vi "Main.vi"(8 "Error In":errorcluster) -> (0 "Error Out":errorcluster)   [LabVIEW 2017, in "Processing.lvlib"]
uses:
  Processing.lvlib
  Controls/Commands [enum].ctl
  File IO/Controls/Params.ctl
  System Control/CTLs/Test params.ctl
  System Control/CTLs/Test Controls.ctl
  System Control/CTLs/Test indicators.ctl
  System Control/CTLs/Test Type.ctl
  Events/Controls/Action Refs [enum].ctl
  System Control/Main controller.lvlib
  Events/Events.lvlib
  File IO/File IO.lvlib
  UI/UI.lvlib
panel:
  in  "Test":T1={"Config"={"Amplification Factor"=2.0, "100% Reflectance Standard"=2.0, "Calculation Method"=enum."Reflectance", "Option to discard new data?"=FALSE, "Mode"=enum."Spectrum", "Number of Averages"=0, "B Test?"=FALSE}, "Indicators"={"DAQ Background Level (V)"=2.0, "A-Test Counter"=2, "B-Test Counter"=2, "Type"=enum."A-Test", "Scope Background Level (Amps)"=2.0, "TAS only?"=FALSE}} {"Config"."Number of Averages" min=0}
  in  "File IO parameters":T5={"Output Folder"=path "C:/Users/Abigail/Documents/Imperial Optical software/Optical Software Code Simplified/Output", "Error file"=path "Error Log.txt", "Config file"=path "Config.ini", "File prefix"="", "Waveform read"={"t0"=timestamp(0 s since 1904-01-01), "dt"=1.0, "Y"=[]}}
  in  "Change state":T6
  out "Standalone":bool=TRUE
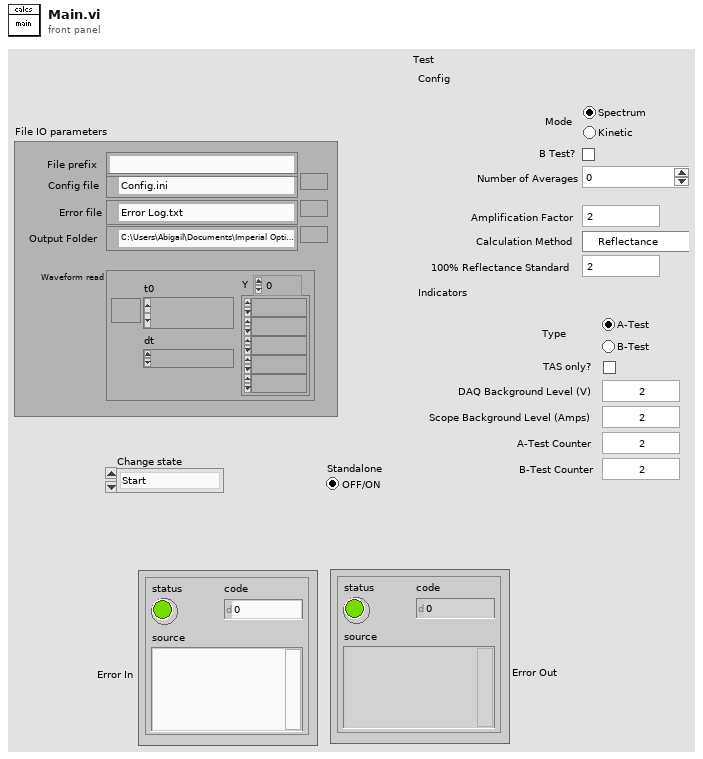
[diagram p1: front panel]
types:
  T1 = typedef "Main controller.lvlib/Test params.ctl" = cluster{"Config":T2, "Indicators":T3}
  T2 = typedef "Main controller.lvlib/Test Controls.ctl" = cluster{"Amplification Factor":dbl, "100% Reflectance Standard":dbl, "Calculation Method":enum16{"Reflectance", "Transmission", "Kubelka-Munk"}, "Option to discard new data?":bool, "Mode":enum32{"Spectrum", "Kinetic"}, "Number of Averages":i32, "B Test?":bool}
  T3 = typedef "Main controller.lvlib/Test indicators.ctl" = cluster{"DAQ Background Level (V)":dbl, "A-Test Counter":i32, "B-Test Counter":i32, "Type":T4, "Scope Background Level (Amps)":dbl, "TAS only?":bool}
  T4 = typedef "Main controller.lvlib/Test Type.ctl" = enum32{"A-Test", "B-Test"}
  T5 = typedef "File IO.lvlib/Params.ctl" = cluster{"Output Folder":path, "Error file":path, "Config file":path, "File prefix":string, "Waveform read":waveform(dbl)}
  T6 = typedef "Processing.lvlib/Commands [enum].ctl" = enum16{"Start", "Stop", "Process waveform", "Scope A-B processing", "DAQ A-B processing", "DAQ-Scope Stitching", "Update Test Info"}
  T7 = enum32{"Bad", "Idle", "Run top level", "Running"}
  T8 = typedef "Events.lvlib/Action Refs [enum].ctl" = enum16{"Init", "Ref", "Kill"}
  T9 = typedef "Events.lvlib/Refs [cluster].ctl" = cluster{"Exit":refnum<user-event>, "Controller":refnum<user-event>, "System Error":refnum<user-event>, "UI":refnum<user-event>, "Example Module":refnum<user-event>, "Shutter":refnum<user-event>, "Monochromator":refnum<user-event>, "DAQ":refnum<user-event>, "Scope":refnum<user-event>, "Processing":refnum<user-event>, "File IO":refnum<user-event>, "Colour wheel":refnum<user-event>}
  T10 = cluster{"Debug Waveform Read":dbl[][], "Waveform name":string}
  T11 = cluster{"File IO":T5, "Filename (A)":string, "Filename (B)":string}
  T12 = cluster{"File IO":T5, "DAQ Filename":string, "Scope Filename":string}
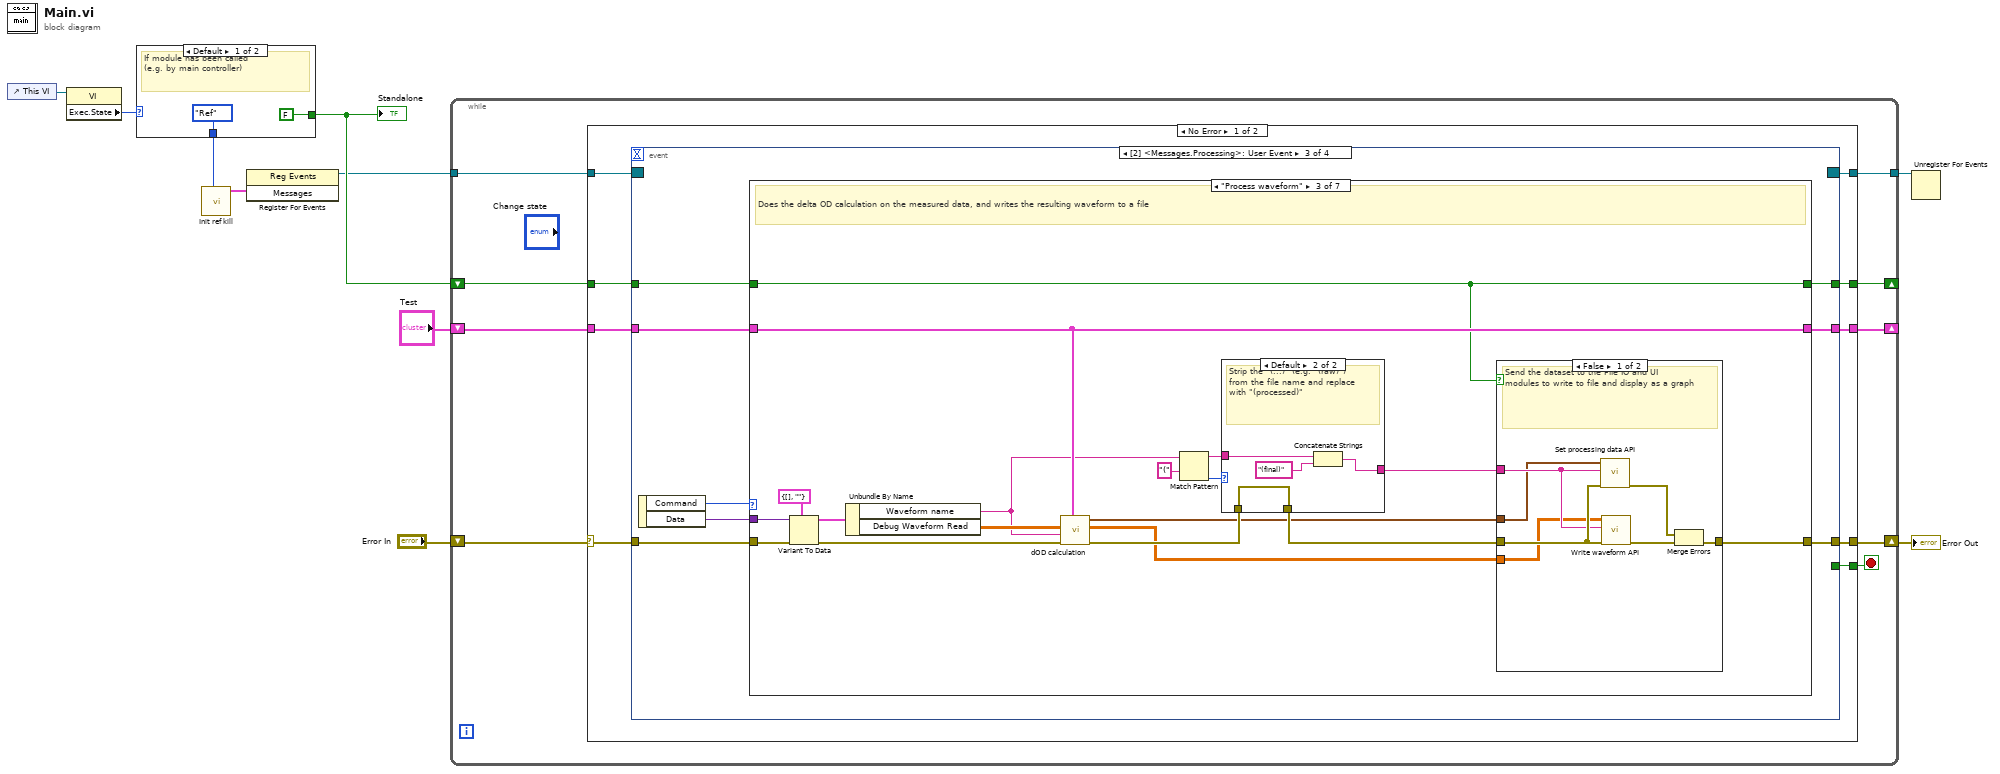
[diagram p0: block diagram]
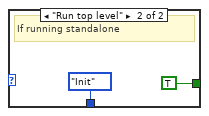
[diagram p2: hidden frame]
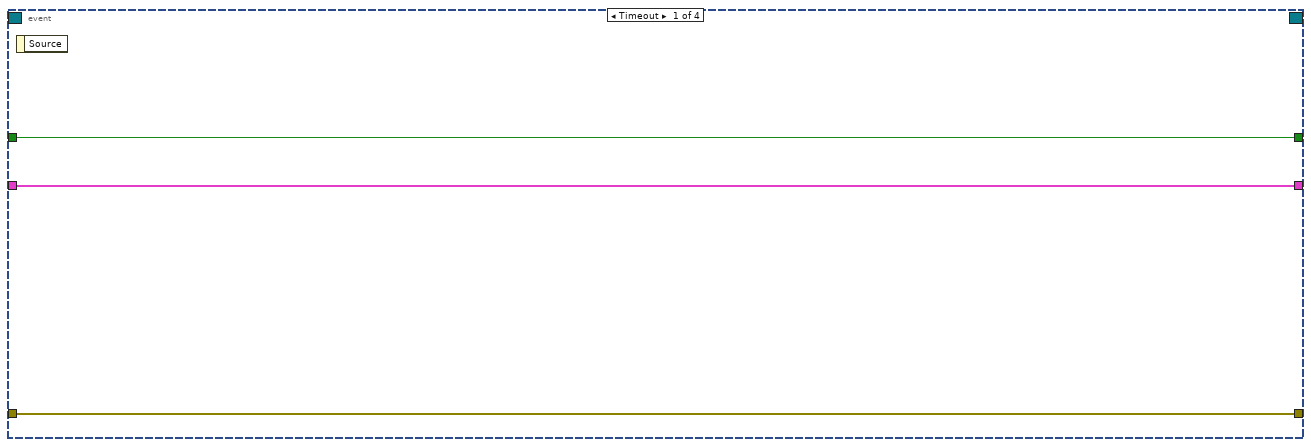
[diagram p3: hidden frame]
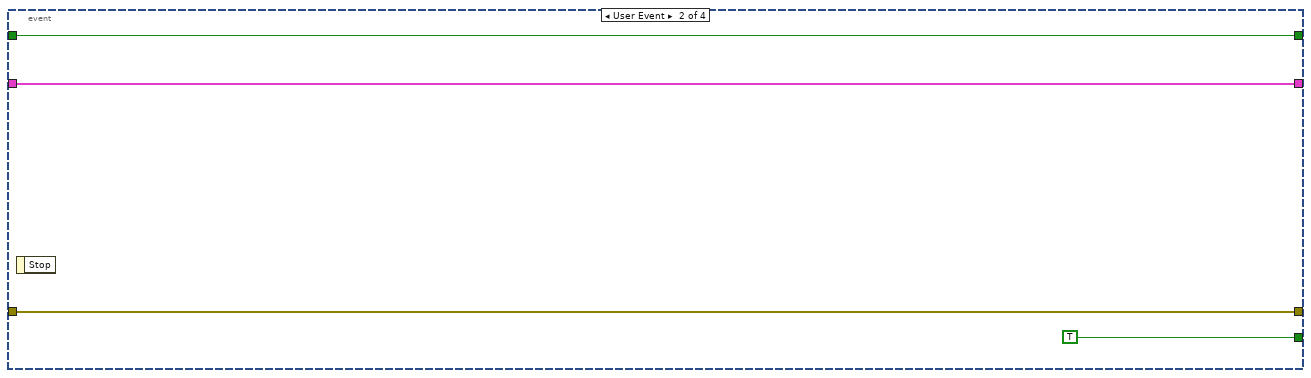
[diagram p4: hidden frame]
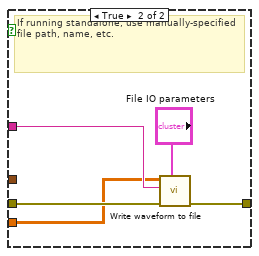
[diagram p7: hidden frame]
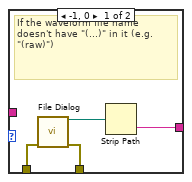
[diagram p8: hidden frame]
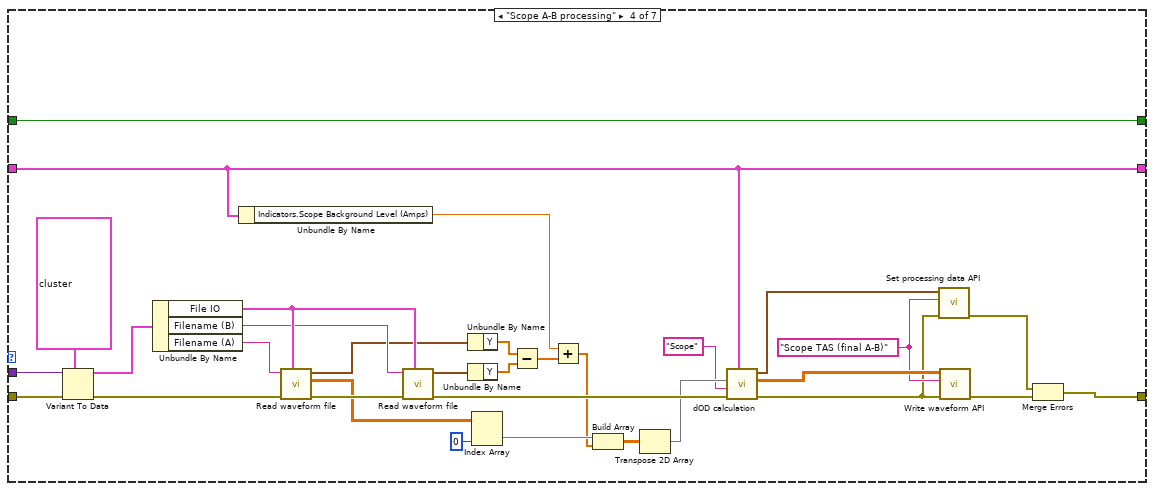
[diagram p9: hidden frame]
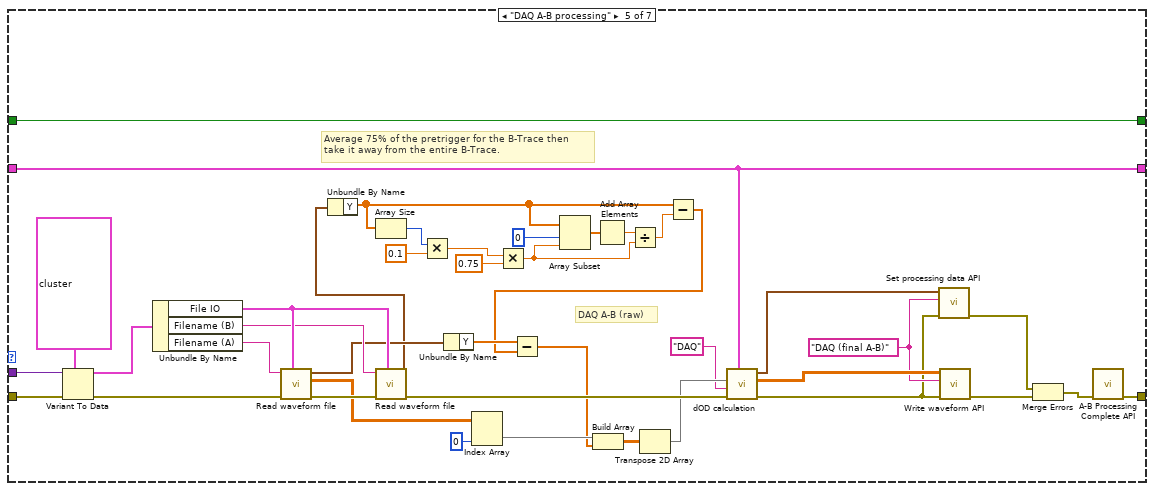
[diagram p10: hidden frame]
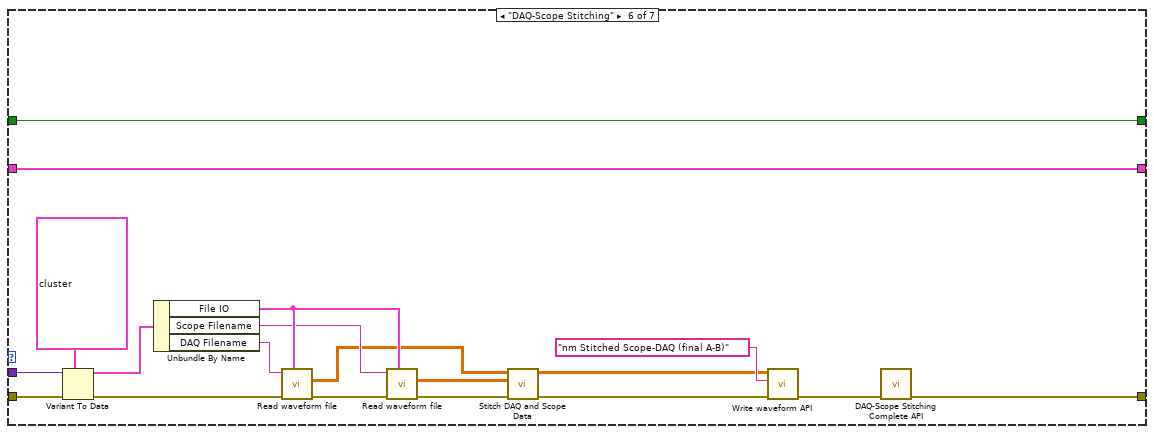
[diagram p11: hidden frame]
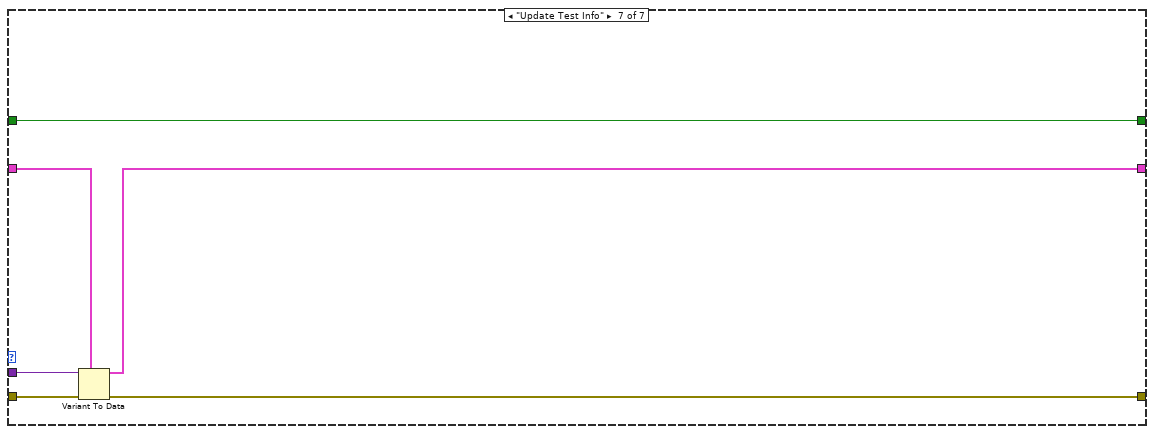
[diagram p12: hidden frame]
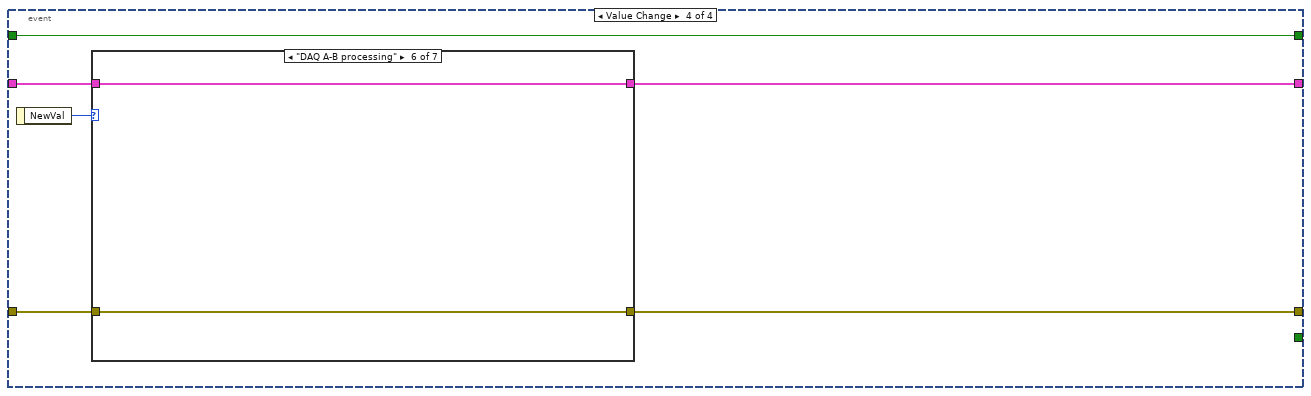
[diagram p13: hidden frame]
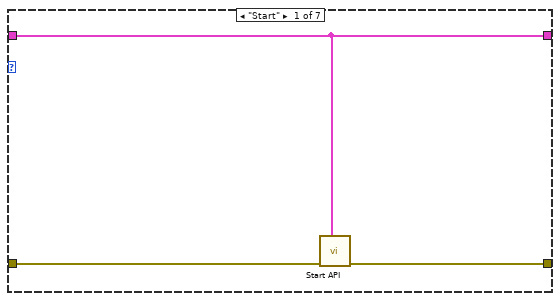
[diagram p14: hidden frame]
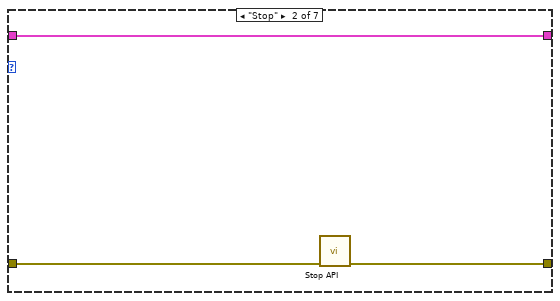
[diagram p15: hidden frame]
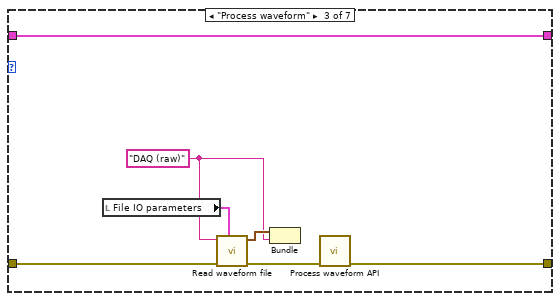
[diagram p16: hidden frame]
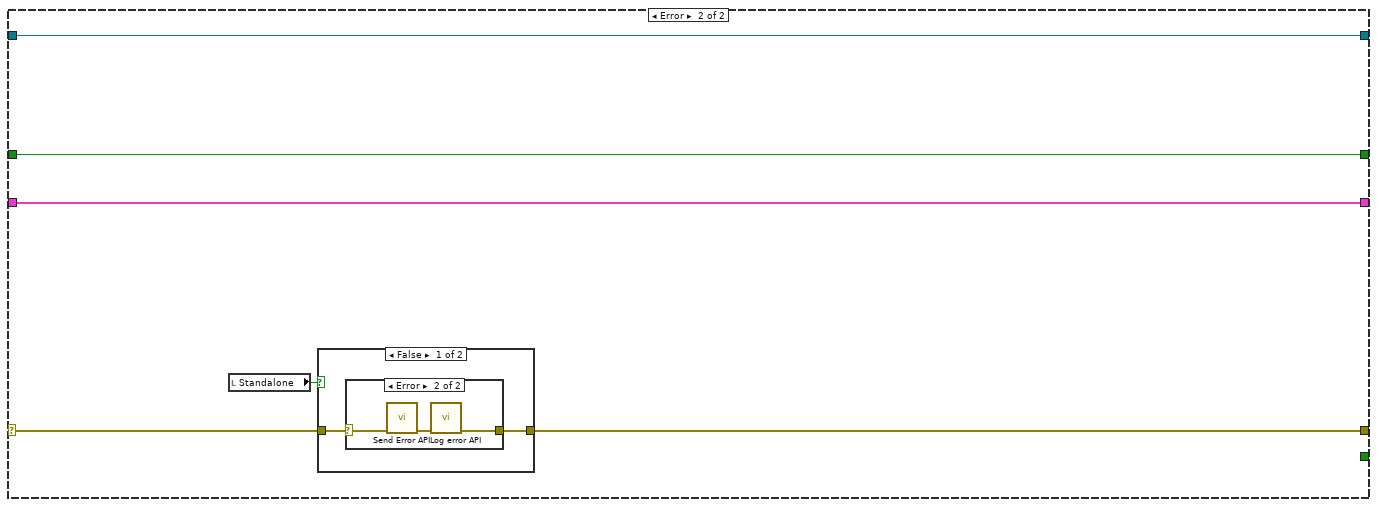
[diagram p20: hidden frame]
diagram:
  n1 = control-ref of="This VI"() -> (w5:refnum<vi>)
  n2 = property class="VI"(reference=w5) -> ("Exec.State"=w4:T7)  [unwired: 1 in, 2 out]
  n3 = case shown="Default" w4 {
    tunnel: [Action_Refs_[enum]."Ref" ("Action") Action_Refs_[enum]."Init" ("Action")] -> w3
    tunnel: [FALSE TRUE] -> w2
    frame Default {
      # "If module has been called\n(e.g. by main controller)"
    }
    frame "Run top level" {
      # "If running standalone"
    }
  }
  "Standalone" <- w2
  n4 = call "Init ref kill.vi"("Action"=w3) -> ("Messages"=w6:T9)  [unwired: 9 in, 1 out]
  n5 = register-events(w6) -> (reference out=w1:refnum<event-registration>)  [unwired: 2 in, 1 out]
  n6 = while {
    tunnel: w1 -> [w23]
    shift-right: [w20] -> _
    shift-left: w2 -> [w19]
    tunnel: [w21] -> w10
    shift-right: [w16] -> w8
    shift-left: "Error In" -> [w15]
    shift-right: [w17] -> _
    shift-left: "Test" -> [w18]
    stop <- w22 stop-if-true
    n7 = case shown="No Error" w15 {
      selector: w15 -> [w24 w222]
      tunnel: w23 -> [w32 w217]
      tunnel: [w31 _] -> w22
      tunnel: [w30 w217] -> w21
      tunnel: [w29 w218] -> w20
      tunnel: w19 -> [w28 w218]
      tunnel: w18 -> [w27 w219]
      tunnel: [w26 w219] -> w17
      tunnel: [w25 w221] -> w16
      frame No Error {
        n8 = event shown="[2] <Messages.Processing>: User Event" {
          selector: w32 -> [_ _ _ _]
          dyn-events: [_ _ _ _] -> w30
          timeout: _ -> [_ _ _ _]
          tunnel: [_ TRUE _ _] -> w31
          tunnel: [w33 w36 w46 w195] -> w29
          tunnel: w28 -> [w33 w36 w45 w195]
          tunnel: w24 -> [w34 w37 w43 w192]
          tunnel: [w34 w37 w42 w191] -> w25
          tunnel: w27 -> [w35 w38 w41 w194]
          tunnel: [w35 w38 w40 w193] -> w26
          event Timeout {
            n9 = event-data() -> ()  [unwired: 1 in, 1 out]
          }
          event User Event {
            n10 = event-data() -> ()  [unwired: 1 in, 1 out]
          }
          event User Event {
            n11 = event-data() -> ("Command"=w47:T6, "Data"=w44:variant)  [unwired: 1 in]
            n12 = case shown="\"Process waveform\"" w47 {
              tunnel: [w49 w52 w59 w123 w164 w183 w189] -> w46
              tunnel: w45 -> [w49 w52 w59 w123 w164 w183 w189]
              tunnel: w44 -> [_ _ w70 w122 w163 w182 w186]
              tunnel: w43 -> [w48 w51 w71 w121 w162 w181 w188]
              tunnel: [w48 w51 w62 w92 w149 w175 w187] -> w42
              tunnel: w41 -> [w50 w53 w63 w94 w137 w178 w185]
              tunnel: [w50 w53 w63 w94 w137 w178 w184] -> w40
              frame "Start" {
                # "Initialise stuff"
              }
              frame "Stop" {
                # "Close stuff"
              }
              frame "Process waveform" {
                # "Does the delta OD calculation on the measured data, and writes the resulting waveform to a file"
                n13 = Variant To Data(error in=w71, type=T10 {"Debug Waveform Read"=[], "Waveform name"=""} ("Waveform + name 2"), Variant=w70) -> (data=w68:T10, error out=w69:errorcluster)
                n14 = Unbundle By Name(w68) -> ("Waveform name"=w54:string, "Debug Waveform Read"=w56:dbl[][])
                n15 = call "dOD calculation.vi"("Test"=w63, "error in"=w69, "Waveform Name"=w54, "Debug Waveform Read In"=w56) -> ("error out"=w64:errorcluster, "Debug Waveform Read Out"=w55:dbl[][], "dOD waveform"=w58:waveform(dbl))  [unwired: 5 in]
                n16 = Match Pattern(string=w54, regular expression="(") -> (before substring=w66:string, offset past match=w65:i32)  [unwired: 1 in, 2 out]
                n17 = case shown="Default" w65 {
                  tunnel: w66 -> [_ w91]
                  tunnel: [w87 w89] -> w60
                  tunnel: w64 -> [w85 w88]
                  tunnel: [w84 w88] -> w61
                  frame -1, 0 {
                    # "If the waveform file name doesn't have \"(...)\" in it (e.g. \"(raw)\")"
                    n18 = call "File Dialog"("error in"=w85) -> ("selected path"=w86:path, "error out"=w84:errorcluster)  [unwired: 11 in, 2 out]
                    n19 = Strip Path(path=w86) -> (name=w87:string)  [unwired: 1 out]
                  }
                  frame Default {
                    # "Strip the \"(...)\" (e.g. \"(raw)\") from the file name and replace with \"(processed)\""
                    n20 = Concatenate Strings(w91, "(final)" ("string")) -> (w89:string)
                  }
                }
                n21 = case shown="False" w59 {
                  tunnel: [w78 w83] -> w62
                  tunnel: w58 -> [w73 _]
                  tunnel: w61 -> [w76 w82]
                  tunnel: w60 -> [w74 w81]
                  tunnel: w55 -> [w72 w79]
                  frame False {
                    # "Send the dataset to the File IO and UI modules to write to file and display as a graph"
                    n22 = call "Set processing data API.vi"("Error In"=w76, "Waveform name"=w74, "Waveform"=w73) -> ("Error Out"=w75:errorcluster)  [unwired: 8 in]
                    n23 = call "Write waveform API.vi"("Error In"=w76, "Waveform name"=w74, "Waveform Data"=w72) -> ("Error Out"=w77:errorcluster)  [unwired: 8 in]
                    n24 = Merge Errors(w75, w77) -> (w78:errorcluster)
                  }
                  frame True {
                    # "If running standalone, use manually-specified file path, name, etc."
                    n25 = call "Write waveform to file.vi"("File IO parameters"="File IO parameters", "error in"=w82, "Dataset name"=w81, "Data"=w79) -> ("error out"=w83:errorcluster)  [unwired: 7 in]
                  }
                }
              }
              frame "Scope A-B processing" {
                w98 = "Scope TAS (final A-B)" ("Waveform name")
                n26 = Variant To Data(error in=w121, type=T11 {"File IO"={"Output Folder"=path "", "Error file"=path "", "Config file"=path "", "File prefix"="", "Waveform read"={"t0"=timestamp(0 s since 1904-01-01), "dt"=1.0, "Y"=[]}}, "Filename (A)"="", "Filename (B)"=""}, Variant=w122) -> (data=w118:T11, error out=w120:errorcluster)
                n27 = Unbundle By Name(w118) -> ("File IO"=w116:T5, "Filename (B)"=w115:string, "Filename (A)"=w114:string)
                n28 = Unbundle By Name(w94) -> ("Indicators.Scope Background Level (Amps)"=w93:dbl)
                n29 = call "Read waveform file.vi"("File IO parameters"=w116, "error in"=w120, "Dataset name"=w114) -> ("error out"=w117:errorcluster, "all rows"=w107:dbl[][], "Waveform"=w113:waveform(dbl))  [unwired: 6 in]
                n30 = call "Read waveform file.vi"("File IO parameters"=w116, "error in"=w117, "Dataset name"=w115) -> ("error out"=w108:errorcluster, "Waveform"=w112:waveform(dbl))  [unwired: 6 in, 1 out]
                n31 = Unbundle By Name(w113) -> ("Y"=w110:dbl[])
                n32 = Unbundle By Name(w112) -> ("Y"=w111:dbl[])
                n33 = Index Array(array=w107, index (col)=0 ("disabled index (col)")) -> (element=w105:dbl[])  [unwired: 1 in]
                n34 = Subtract(x=w110, y=w111) -> (x-y=w109:dbl[])
                n35 = Add(x=w93, y=w109) -> (x+y=w104:dbl[])
                n36 = Build Array(w105, w104) -> (w103:dbl[][])
                n37 = Transpose 2D Array(2D array=w103) -> (transposed array=w102:dbl[][])
                n38 = call "dOD calculation.vi"("Test"=w94, "error in"=w108, "Waveform Name"="Scope", "Debug Waveform Read In"=w102) -> ("error out"=w97:errorcluster, "Debug Waveform Read Out"=w99:dbl[][], "dOD waveform"=w100:waveform(dbl))  [unwired: 5 in]
                n39 = call "Set processing data API.vi"("Error In"=w97, "Waveform name"=w98, "Waveform"=w100) -> ("Error Out"=w96:errorcluster)  [unwired: 8 in]
                n40 = call "Write waveform API.vi"("Error In"=w97, "Waveform name"=w98, "Waveform Data"=w99) -> ("Error Out"=w95:errorcluster)  [unwired: 8 in]
                n41 = Merge Errors(w96, w95) -> (w92:errorcluster)
              }
              frame "DAQ A-B processing" {
                w142 = "DAQ (final A-B)" ("Waveform name")
                # "Average 75% of the pretrigger for the B-Trace then \ntake it away from the entire B-Trace."
                # "DAQ A-B (raw)"
                n42 = Variant To Data(error in=w162, type=T11 {"File IO"={"Output Folder"=path "", "Error file"=path "", "Config file"=path "", "File prefix"="", "Waveform read"={"t0"=timestamp(0 s since 1904-01-01), "dt"=1.0, "Y"=[]}}, "Filename (A)"="", "Filename (B)"=""}, Variant=w163) -> (data=w159:T11, error out=w161:errorcluster)
                n43 = Unbundle By Name(w159) -> ("File IO"=w157:T5, "Filename (B)"=w156:string, "Filename (A)"=w155:string)
                n44 = call "Read waveform file.vi"("File IO parameters"=w157, "error in"=w161, "Dataset name"=w155) -> ("error out"=w158:errorcluster, "all rows"=w151:dbl[][], "Waveform"=w154:waveform(dbl))  [unwired: 6 in]
                n45 = call "Read waveform file.vi"("File IO parameters"=w157, "error in"=w158, "Dataset name"=w156) -> ("error out"=w152:errorcluster, "Waveform"=w125:waveform(dbl))  [unwired: 6 in, 1 out]
                n46 = Unbundle By Name(w125) -> ("Y"=w135:dbl[])
                n47 = Array Size(array=w135) -> (size(s)=w134:i32)
                n48 = Multiply(x=w134, y=0.1) -> (x*y=w133:dbl)
                n49 = Unbundle By Name(w154) -> ("Y"=w153:dbl[])
                n50 = Index Array(array=w151, index (col)=0 ("disabled index (col)")) -> (element=w148:dbl[])  [unwired: 1 in]
                n51 = Multiply(x=w133, y=0.75) -> (x*y=w132:dbl)
                n52 = Array Subset(array=w135, index=0, length=w132) -> (w131:dbl[])
                n53 = Add Array Elements(numeric array=w131) -> (sum=w130:dbl)
                n54 = Divide(x=w130, y=w132) -> (x/y=w129:dbl)
                n55 = Subtract(x=w135, y=w129) -> (x-y=w124:dbl[])
                n56 = Subtract(x=w153, y=w124) -> (x-y=w136:dbl[])
                n57 = Build Array(w148, w136) -> (w147:dbl[][])
                n58 = Transpose 2D Array(2D array=w147) -> (transposed array=w146:dbl[][])
                n59 = call "dOD calculation.vi"("Test"=w137, "error in"=w152, "Waveform Name"="DAQ", "Debug Waveform Read In"=w146) -> ("error out"=w141:errorcluster, "Debug Waveform Read Out"=w143:dbl[][], "dOD waveform"=w144:waveform(dbl))  [unwired: 5 in]
                n60 = call "Set processing data API.vi"("Error In"=w141, "Waveform name"=w142, "Waveform"=w144) -> ("Error Out"=w140:errorcluster)  [unwired: 8 in]
                n61 = call "Write waveform API.vi"("Error In"=w141, "Waveform name"=w142, "Waveform Data"=w143) -> ("Error Out"=w139:errorcluster)  [unwired: 8 in]
                n62 = Merge Errors(w140, w139) -> (w138:errorcluster)
                n63 = call "A-B Processing Complete API.vi"("Error In"=w138) -> ("Error Out"=w149:errorcluster)  [unwired: 10 in]
              }
              frame "DAQ-Scope Stitching" {
                n64 = Variant To Data(error in=w181, type=T12 {"File IO"={"Output Folder"=path "", "Error file"=path "", "Config file"=path "", "File prefix"="", "Waveform read"={"t0"=timestamp(0 s since 1904-01-01), "dt"=1.0, "Y"=[]}}, "DAQ Filename"="", "Scope Filename"=""}, Variant=w182) -> (data=w179:T12, error out=w174:errorcluster)
                n65 = Unbundle By Name(w179) -> ("File IO"=w172:T5, "Scope Filename"=w170:string, "DAQ Filename"=w171:string)
                n66 = call "Read waveform file.vi"("File IO parameters"=w172, "error in"=w174, "Dataset name"=w171) -> ("error out"=w173:errorcluster, "all rows"=w167:dbl[][])  [unwired: 6 in, 1 out]
                n67 = call "Read waveform file.vi"("File IO parameters"=w172, "error in"=w173, "Dataset name"=w170) -> ("error out"=w169:errorcluster, "all rows"=w166:dbl[][])  [unwired: 6 in, 1 out]
                n68 = call "Stitch DAQ and Scope Data.vi"("error in (no error)"=w169, "Scope Ch1 (final A-B)"=w166, "DAQ DOD (final)"=w167) -> ("error out"=w168:errorcluster, "data & time array"=w165:dbl[][])  [unwired: 7 in]
                n69 = call "Write waveform API.vi"("Error In"=w168, "Waveform name"="nm Stitched Scope-DAQ (final A-B)", "Waveform Data"=w165) -> ("Error Out"=w176:errorcluster)  [unwired: 8 in]
                n70 = call "DAQ-Scope Stitching Complete API.vi"("Error In"=w176) -> ("Error Out"=w175:errorcluster)  [unwired: 10 in]
              }
              frame "Update Test Info" {
                n71 = Variant To Data(error in=w188, type=w185, Variant=w186) -> (data=w184:T1, error out=w187:errorcluster)
              }
            }
          }
          event Value Change {
            n72 = event-data() -> ("NewVal"=w190:T6)  [unwired: 1 in]
            n73 = case shown="\"DAQ A-B processing\"" w190 {
              tunnel: w194 -> [w196 w201 w207 w210 w212 w214 w216]
              tunnel: [w196 w201 w207 w210 w212 w214 w216] -> w193
              tunnel: [w197 w199 w208 w209 w211 w213 w215] -> w191
              tunnel: w192 -> [w198 w200 w206 w209 w211 w213 w215]
              frame "Start" {
                n74 = call "Start API.vi"("Test"=w196, "Error In"=w198) -> ("Error Out"=w197:errorcluster)  [unwired: 9 in]
              }
              frame "Stop" {
                n75 = call "Stop API.vi"("Error In"=w200) -> ("Error Out"=w199:errorcluster)  [unwired: 10 in]
              }
              frame "Process waveform" {
                w203 = "DAQ (raw)" ("Dataset name")
                n76 = local read "File IO parameters"() -> (w202:T5)
                n77 = call "Read waveform file.vi"("File IO parameters"=w202, "error in"=w206, "Dataset name"=w203) -> ("error out"=w205:errorcluster, "Waveform"=w204:waveform(dbl))  [unwired: 6 in, 1 out]
                n78 = Bundle("Waveform"=w204, "Dataset name"=w203) -> ()  [unwired: 1 in, 1 out]
                n79 = call "Process waveform API.vi"("Error In"=w205) -> ("Error Out"=w208:errorcluster)  [unwired: 10 in]
              }
              frame "DAQ-Scope Stitching" {
              }
              frame "Scope A-B processing" {
              }
              frame "DAQ A-B processing" {
              }
              frame "Update Test Info" {
              }
            }
          }
        }
      }
      frame Error {
        n80 = local read "Standalone"() -> (w220:bool)
        n81 = case shown="False" w220 {
          tunnel: [w224 _] -> w221
          tunnel: w222 -> [w223 w229]
          frame False {
            n82 = case shown="Error" w223 {
              selector: w223 -> [w225 w227]
              tunnel: [w225 w228] -> w224
              frame No Error {
              }
              frame Error {
                n83 = call "Send Error API.vi"("Error Cluster"=w227) -> ("Error Out"=w226:errorcluster)  [unwired: 10 in]
                n84 = call "Log error API.vi"("Error In"=w226) -> ("Error Out"=w228:errorcluster)  [unwired: 10 in]
              }
            }
          }
          frame True {
            n85 = call <vilib>:"Simple Error Handler.vi"("error in (no error)"=w229) -> ()  [unwired: 4 in, 5 out]
          }
        }
      }
    }
  }
  "Error Out" <- w8
  n86 = Unregister For Events(event registration refnum=w10) -> ()  [unwired: 1 in, 1 out]
